vi "KH7008 Set Channel.vi"(8 "error in (no error)":errorcluster, 10 "Channel Parameters":T1={"Channel"=enum."Channel 2", "Gain"=enum."10x", "Bandwidth Filter"=enum."ON", "Shunt Resistor"=enum."50 Ohms", "Coupling"=enum."DC", "Input Config"=enum."Differential"}, 11 "VISA Refnum in":refnum<visa-resource-name>="COM1") -> (0 "error out":errorcluster, 3 "VISA Refnum out":refnum<visa-resource-name>)   [LabVIEW 2019, in "Instrument.KH7008.lvclass"]
uses:
  Instrument.KH7008.lvclass
  typedefs/SetAll-Cluster.ctl
  typedefs/Channel-Enum.ctl
  typedefs/Gain-Enum.ctl
  typedefs/Filter-Enum.ctl
  typedefs/Shunt-Enum.ctl
  typedefs/Coupling-Enum.ctl
  typedefs/Input Configuration-Enum.ctl
panel:
  out "Response":string
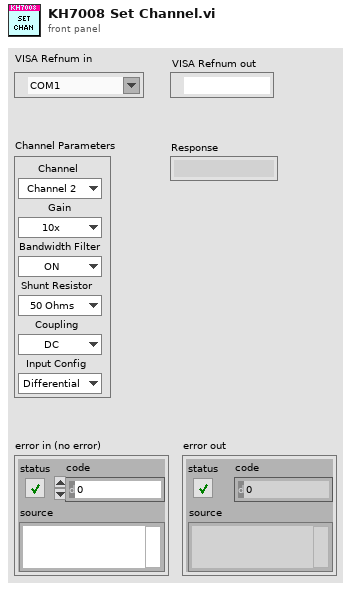
[diagram p1: front panel]
types:
  T1 = typedef "Instrument.KH7008.lvclass/SetAll-Cluster.ctl" = cluster{"Channel":T2, "Gain":T3, "Bandwidth Filter":T4, "Shunt Resistor":T5, "Coupling":T6, "Input Config":T7}
  T2 = typedef "Instrument.KH7008.lvclass/Channel-Enum.ctl" = enum16{"Channel 1", "Channel 2", "Channel 3", "Channel 4", "Channel 5", "Channel 6", "Channel 7", "Channel 8"}
  T3 = typedef "Instrument.KH7008.lvclass/Gain-Enum.ctl" = enum16{"1x", "10x", "100x", "1000x"}
  T4 = typedef "Instrument.KH7008.lvclass/Filter-Enum.ctl" = enum16{"OFF", "ON"}
  T5 = typedef "Instrument.KH7008.lvclass/Shunt-Enum.ctl" = enum16{"Open", "50 Ohms", "500 Ohms", "5k Ohms", "50k Ohms", "10M Ohm"}
  T6 = typedef "Instrument.KH7008.lvclass/Coupling-Enum.ctl" = enum16{"AC", "DC"}
  T7 = typedef "Instrument.KH7008.lvclass/Input Configuration-Enum.ctl" = enum16{"Ground", "SE+ (-gnd)", "SE- (+gnd)", "Differential"}
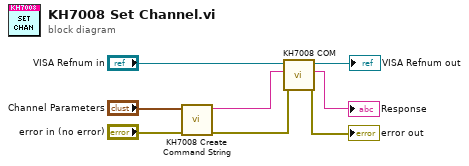
[diagram p0: block diagram]
diagram:
  n1 = call "KH7008 Create Command String.vi"("error in (no error)"="error in (no error)", "Channel Parameters"="Channel Parameters") -> ("error out"=w4:errorcluster, "Command string"=w1:string)  [unwired: 8 in]
  n2 = call "KH7008 COM.vi"("error in (no error)"=w4, "Command"=w1, "VISA Refnum in"="VISA Refnum in") -> ("error out"=→"error out":errorcluster, "Response"=→"Response":string, "VISA Refnum out"=→"VISA Refnum out":refnum<visa-resource-name>)  [unwired: 6 in]
